vi "front_panel.vi"() -> ()   [LabVIEW 2026]
uses:
  <vilib>/OpenLvVision/OpenLvVision_Image/Management/TypeDef/OLV ImageType.ctl
  <vilib>/OpenLvVision/OpenLvVision_OpenCv/VideoIO/VideoCapture/Public/Open/OLV VideoCapture Open_Device.vi
  <vilib>/OpenLvVision/OpenLvVision_Image/DataAccess/ImageToArray/OLV ImageColorU32ToArray.vi
  <vilib>/OpenLvVision/OpenLvVision_Image/DataAccess/ArrayToImage/OLV ArrayColorU32ToImage.vi
  <vilib>/OpenLvVision/OpenLvVision_OpenCv/VideoIO/VideoCapture/OLV VideoCapture.lvclass
  <vilib>/OpenLvVision/OpenLvVision_Image/DataAccess/OLV DataAccess.lvlib
  <vilib>/OpenLvVision/OpenLvVision_Image/File/OLV File.lvlib
  <vilib>/OpenLvVision/OpenLvVision_Image/Management/OLV Management.lvlib
panel:
  in  "Space":bool
  in  "EmptyText":bool
  in  "Speak":bool
  out "Text":string
  in  "Hand":bool
  in  "Next_letter":bool
  in  "Input":bool
  in  "Filename":string
  out "Image":T1(plugin-control)
  out "Prediction":string
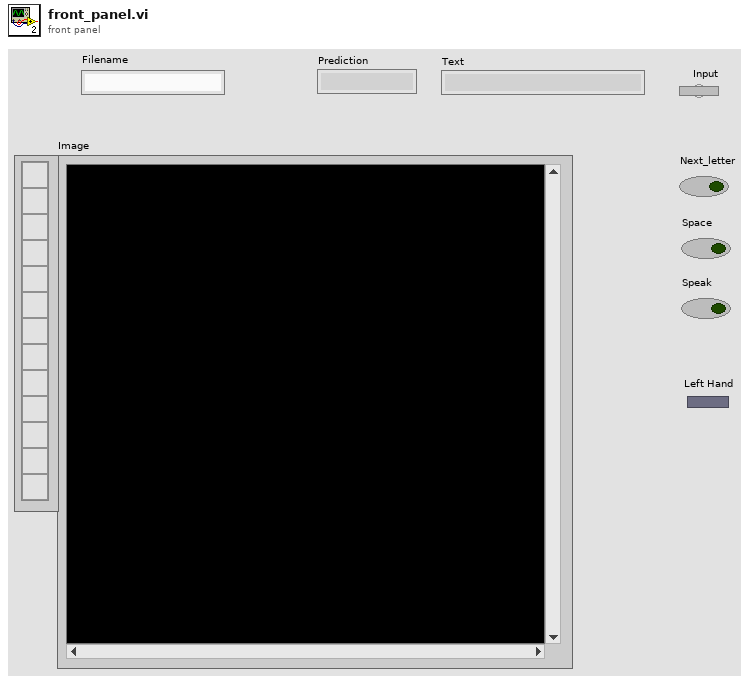
[diagram p1: front panel]
types:
  T1 = typedef "IMAQ Image.ctl" = refnum<image>
  T2 = typedef "OLV OpenLvVision_Image.lvlib/OLV Management.lvlib/OLV ImageType.ctl" = enum16{"Mono U8", "Mono U16", "Mono I16", "Mono SGL", "Color U32", "Color U64", "Complex CSG"}
  T3 = typedef "OLV OpenLvVision_Image.lvlib/OLV Management.lvlib/OLV Image.ctl" = refnum<image>
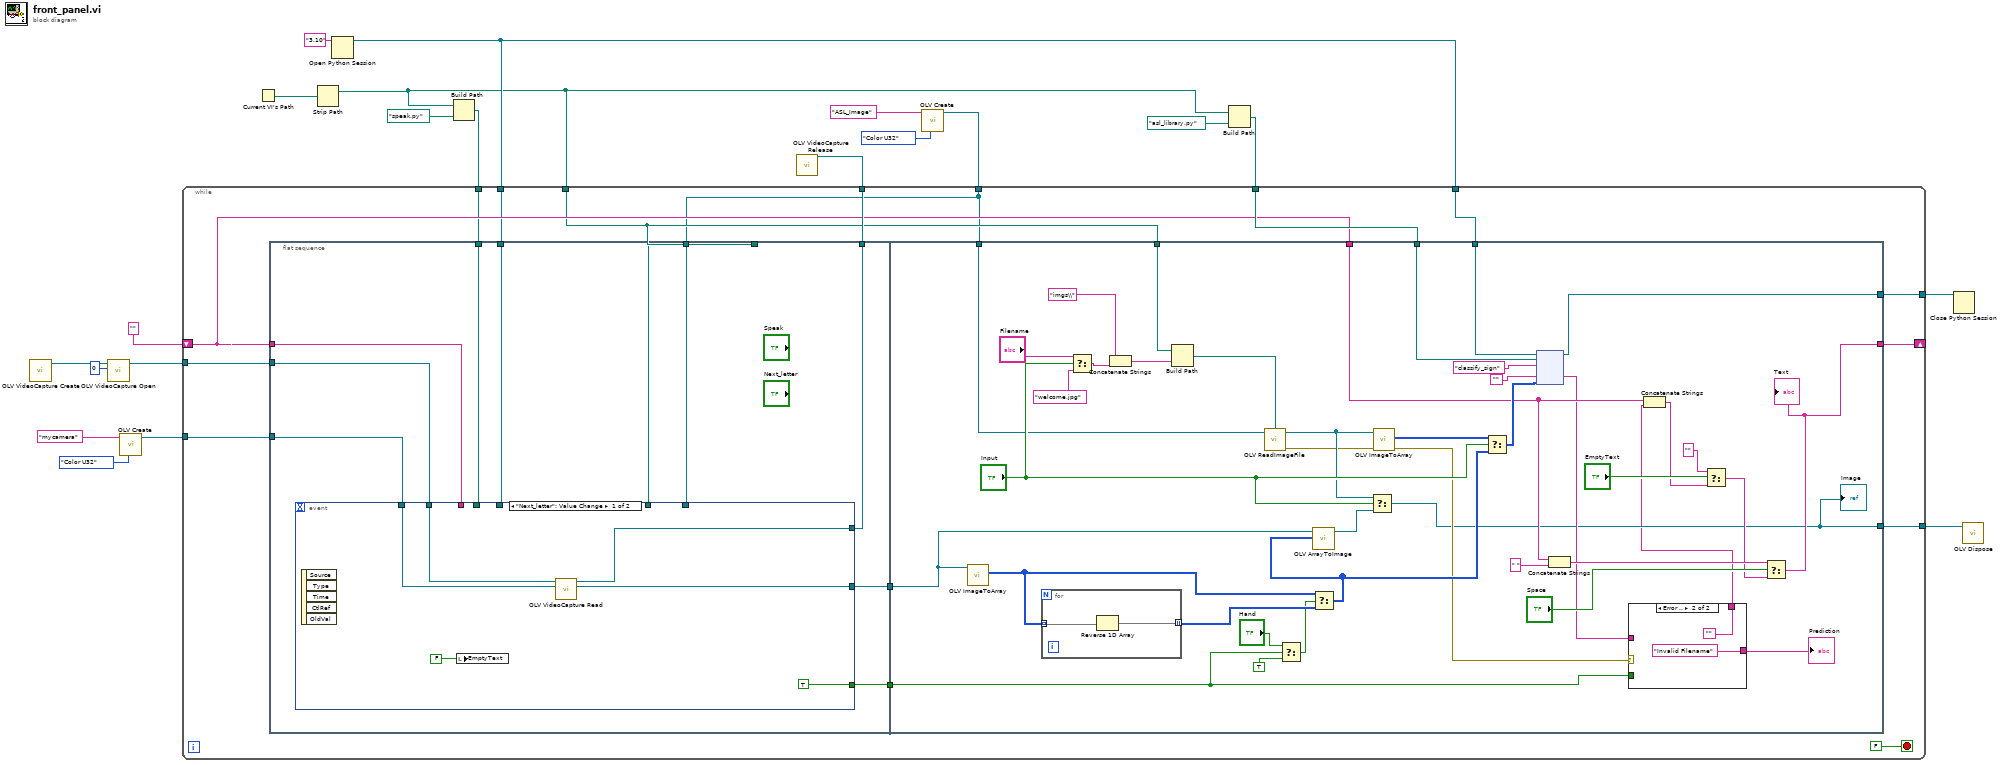
[diagram p0: block diagram]
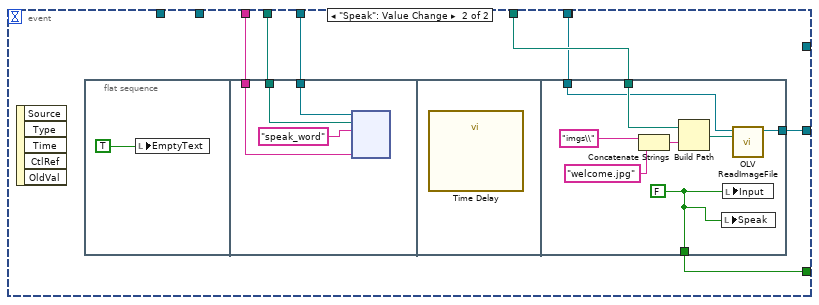
[diagram p2: hidden frame]
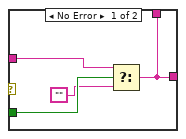
[diagram p3: hidden frame]
diagram:
  n1 = call <vilib>:"OLV VideoCapture Create.vi"() -> ("VideoCapture out"=w4:refnum<class "OLV VideoCapture.lvclass">)  [unwired: 10 in, 1 out]
  n2 = call-poly <vilib>:"OLV VideoCapture Open.vi"("index"=0, "VideoCapture in"=w4) -> ("VideoCapture out"=w5:refnum<class "OLV VideoCapture.lvclass">)  [unwired: 7 in, 2 out]
  n3 = call <vilib>:"OLV Create.vi"("Image Type"=OLV_ImageType."Color U32", "Image Name"="mycamera") -> ("Image Reference Out"=w6:T3)  [unwired: 8 in, 1 out]
  n4 = Current VI's Path() -> (path=w15:path)
  n5 = Strip Path(path=w15) -> (stripped path=w12:path)  [unwired: 1 out]
  n6 = Open Python Session(python version="3.10" ("Python version")) -> (session out=w16:refnum<k35>)  [unwired: 2 in, 1 out]
  n7 = Build Path(base path=w12, name or relative path=path "speak.py" ("module path")) -> (appended path=w13:path)
  n8 = call <vilib>:"OLV Create.vi"("Image Type"=OLV_ImageType."Color U32", "Image Name"="ASL_Image") -> ("Image Reference Out"=w9:T3)  [unwired: 8 in, 1 out]
  n9 = Build Path(base path=w12, name or relative path=path "asl_library.py" ("module path")) -> (appended path=w18:path)
  n10 = while {
    tunnel: w5 -> [w37]
    tunnel: [w36] -> w21
    tunnel: [w35] -> w11
    tunnel: w16 -> [w34]
    tunnel: w18 -> [w33]
    tunnel: w12 -> [w28]
    tunnel: w9 -> [w27]
    shift-right: [w31] -> _
    shift-left: "" -> [w30]
    tunnel: w16 -> [w29]
    tunnel: w13 -> [w26]
    tunnel: [w23] -> w10
    tunnel: w6 -> [w22]
    stop <- FALSE stop-if-true
    n11 = flat-sequence {
      tunnel: w37 -> [w47]
      tunnel: [w46] -> w35
      tunnel: w30 -> [w45]
      tunnel: w29 -> [w44]
      tunnel: w28 -> [w43]
      tunnel: w27 -> [w42]
      tunnel: w26 -> [w40]
      tunnel: [w41] -> w25
      tunnel: [w39] -> w24
      tunnel: w22 -> [w38]
      tunnel: [w109] -> w36
      tunnel: w34 -> [w108]
      tunnel: w33 -> [w107]
      tunnel: w28 -> [w106]
      tunnel: w27 -> [w81]
      tunnel: w30 -> [w99]
      tunnel: [w91] -> w31
      tunnel: w25 -> [w93]
      tunnel: w24 -> [w83]
      tunnel: [w76] -> w23
      frame #0 {
        n12 = event shown="[0] \"Next_letter\": Value Change" {
          selector: _ -> [_ _]
          dyn-events: _ -> [_ _]
          timeout: _ -> [_ _]
          tunnel: [w51 _] -> w46
          tunnel: w47 -> [w52 _]
          tunnel: w45 -> [_ w57]
          tunnel: w44 -> [_ w58]
          tunnel: w43 -> [_ w60]
          tunnel: w42 -> [w54 w59]
          tunnel: w40 -> [_ w61]
          tunnel: [w54 _] -> _
          tunnel: [TRUE ("Input") w56] -> w41
          tunnel: [w49 w55] -> w39
          tunnel: w38 -> [w50 _]
          event "Next_letter": Value Change {
            n13 = event-data() -> ()  [unwired: 1 in, 5 out]
            n14 = local write "EmptyText"(FALSE ("Speak")) -> ()
            n15 = call <vilib>:"OLV VideoCapture Read.vi"("Image"=w50, "VideoCapture in"=w52) -> ("Image out"=w49:T1, "VideoCapture out"=w51:refnum<class "OLV VideoCapture.lvclass">)  [unwired: 6 in, 2 out]
          }
          event "Speak": Value Change {
            n16 = event-data() -> ()  [unwired: 1 in, 5 out]
            n17 = flat-sequence {
              tunnel: w61 -> [w66]
              tunnel: w57 -> [w64]
              tunnel: w58 -> [w63]
              tunnel: w60 -> [w71]
              tunnel: w59 -> [w67]
              tunnel: [w70] -> w56
              tunnel: [w68] -> w55
              frame #0 {
                n18 = local write "EmptyText"(TRUE ("Ready_to_Speak")) -> ()
              }
              frame #1 {
                n19 = node(w63, w66, "speak_word" ("function name"), w64) -> ()  [unwired: 4 in, 4 out]
              }
              frame #2 {
                n20 = call "Time Delay"() -> ()  [unwired: 11 in, 1 out]
              }
              frame #3 {
                w70 = FALSE ("Input")
                n21 = Concatenate Strings("imgs\\" ("string"), "welcome.jpg" ("string")) -> (w74:string)
                n22 = Build Path(base path=w71, name or relative path=w74) -> (appended path=w69:path)
                n23 = local write "Speak"(w70) -> ()
                n24 = local write "Input"(w70) -> ()
                n25 = call <vilib>:"OLV ReadImageFile.vi"("File Path"=w69, "Image Reference In"=w67) -> ("Image Reference Out"=w68:T3)  [unwired: 5 in, 4 out]
              }
            }
          }
        }
      }
      frame #1 {
        n26 = call-poly <vilib>:"OLV ImageToArray.vi"("Image Reference In"=w83) -> ("Pixel"=w86:u32[][])  [unwired: 8 in, 2 out]
        n27 = for {
          tunnel: w86 -> [w123] mode=indexing
          tunnel: [w122] -> w110 mode=indexing
          n28 = Reverse 1D Array(array=w123) -> (reversed array=w122:u32[])
        }
        n29 = Select(t="Filename", s="Input", f="welcome.jpg") -> (s? t:f=w98:string)
        n30 = Concatenate Strings("imgs\\" ("string"), w98) -> (w115:string)
        n31 = Build Path(base path=w106, name or relative path=w115) -> (appended path=w82:path)
        n32 = call <vilib>:"OLV ReadImageFile.vi"("File Path"=w82, "Image Reference In"=w81) -> ("error out"=w78:errorcluster, "Image Reference Out"=w80:T3)  [unwired: 5 in, 3 out]
        n33 = Select(t="Hand", s=w93, f=TRUE) -> (s? t:f=w92:bool)
        n34 = Select(t=w86, s=w92, f=w110) -> (s? t:f=w84:u32[][])
        n35 = call-poly <vilib>:"OLV ArrayToImage.vi"("Pixel"=w84, "Image Reference In"=w83) -> ("Image Reference Out"=w85:T3)  [unwired: 8 in, 1 out]
        n36 = Select(t=w80, s="Input", f=w85) -> (s? t:f=w76:T3)
        "Image" <- w76
        n37 = call-poly <vilib>:"OLV ImageToArray.vi"("error in"=w78, "Image Reference In"=w80) -> ("error out"=w77:errorcluster, "Pixel"=w79:u32[][])  [unwired: 7 in, 1 out]
        n38 = Select(t=w79, s="Input", f=w84) -> (s? t:f=w111:u32[][])
        n39 = node(w108, w107, "classify_sign" ("function name"), "", w111) -> (w109:refnum<k35>, w94:string)  [unwired: 2 in, 3 out]
        n40 = Concatenate Strings(w99, " " ("string")) -> (w101:string)
        n41 = case shown="Error .." w77 {
          tunnel: w93 -> [w119 _]
          tunnel: w94 -> [w118 _]
          tunnel: [w116 "Invalid Filename"] -> w87
          tunnel: [w116 ""] -> w75
          frame No Error {
            n42 = Select(t=w118, s=w119, f="") -> (s? t:f=w116:string)
          }
          frame Error {
          }
        }
        "Prediction" <- w87
        n43 = Concatenate Strings(w99, w75) -> (w102:string)
        n44 = Select(t="", s="EmptyText", f=w102) -> (s? t:f=w90:string)
        n45 = Select(t=w101, s="Space", f=w90) -> (s? t:f=w91:string)
        "Text" <- w91
      }
    }
  }
  n46 = call <vilib>:"OLV VideoCapture Release.vi"("VideoCapture in"=w11) -> ()  [unwired: 9 in, 2 out]
  n47 = Close Python Session(session in=w21) -> ()  [unwired: 1 in, 1 out]
  n48 = call <vilib>:"OLV Dispose.vi"("Image Reference In"=w10) -> ()  [unwired: 10 in, 1 out]
